vi "Remove Single Wheel from Steering Frame by Name.vi"(8 "error in (no error)":errorcluster, 10 "wheel name":string, 11 "steering frame in":refnum<class "NI_Robotics_Steering Frame.lvclass">) -> (0 "error out":errorcluster, 1 "found?":bool, 2 "removed wheel":refnum<class "NI_Robotics_Wheel.lvclass">, 3 "steering frame out":refnum<class "NI_Robotics_Steering Frame.lvclass">, 4 "frame angle (rad)":dbl, 5 "y position":dbl, 7 "x position":dbl)   [LabVIEW 2017, in "NI_Robotics_Steering Frame.lvclass"]
doc: "Removes the wheel or wheels you specify from <B>steering frame in</B>. You must manually select the polymorphic instance to use."
uses:
  <vilib>/robotics/Steering/Steering Frame/NI_Robotics_Steering Frame.lvclass
  <vilib>/robotics/Steering/Wheel/NI_Robotics_Wheel.lvclass
  <vilib>/robotics/Steering/Steering Frame/NI_Robotics_Steering Frame.lvclass/NI_Robotics_Steering Frame.ctl
  <vilib>/robotics/Steering/Wheel/NI_Robotics_Wheel.lvclass/NI_Robotics_Wheel.ctl
  <vilib>/robotics/Steering/Steering Frame/Get Indexes of Multiple Wheels from Names.vi
  <vilib>/robotics/Steering/Wheel/Get Wheel Name.vi
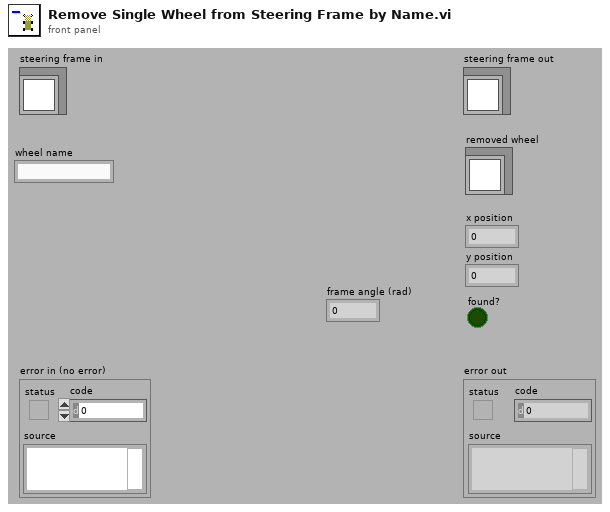
[diagram p1: front panel]
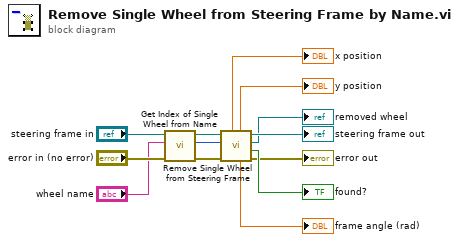
[diagram p0: block diagram]
diagram:
  n1 = call <vilib>:"Get Index of Single Wheel from Name.vi"("error in (no error)"="error in (no error)", "wheel name"="wheel name", "steering frame in"="steering frame in") -> ("error out"=w9:errorcluster, "index"=w8:i32, "steering frame out"=w10:refnum<class "NI_Robotics_Steering Frame.lvclass">)  [unwired: 5 in, 1 out]
  n2 = call <vilib>:"Remove Single Wheel from Steering Frame.vi"("error in (no error)"=w9, "wheel index"=w8, "steering frame in"=w10) -> ("error out"=→"error out":errorcluster, "found?"=→"found?":bool, "removed wheel"=→"removed wheel":refnum<class "NI_Robotics_Wheel.lvclass">, "steering frame out"=→"steering frame out":refnum<class "NI_Robotics_Steering Frame.lvclass">, "frame angle (rad)"=→"frame angle (rad)":dbl, "y position"=→"y position":dbl, "x position"=→"x position":dbl)  [unwired: 2 in]
